vi "ReadXmlFile.vi"() -> ()   [LabVIEW 2018]
uses:
  <vilib>/xml/Load XML File.vi
  <vilib>/xml/Close Reference(Node).vi
  <vilib>/xml/NI_XML.lvlib
panel:
  out "数组":string[](array[string])
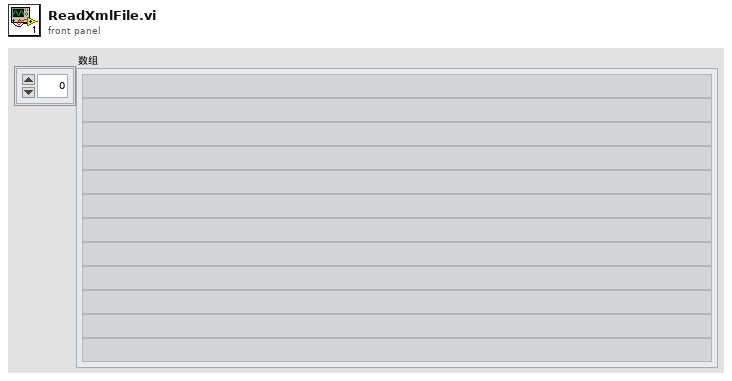
[diagram p1: front panel]
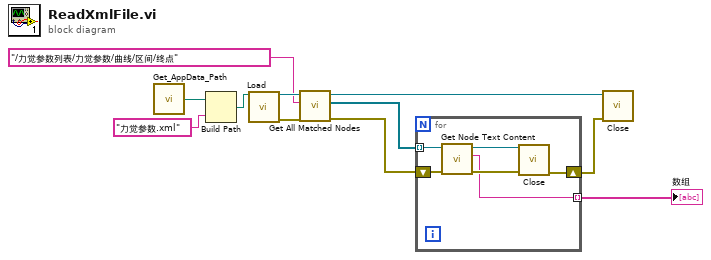
[diagram p0: block diagram]
diagram:
  n1 = call "Get_AppData_Path.vi"() -> ("path"=w7:path)  [unwired: 1 in]
  n2 = Build Path(base path=w7, name or relative path="力觉参数.xml") -> (appended path=w5:path)
  n3 = call-poly <vilib>:"Load.vi"("path to XML document"=w5) -> ("DOM document out"=w11:refnum<k20>, "error out"=w3:errorcluster)  [unwired: 12 in, 1 out]
  n4 = call <vilib>:"Get All Matched Nodes.vi"("error in (no error)"=w3, "XPath expression"="/力觉参数列表/力觉参数/曲线/区间/终点", "node in"=w11) -> ("error out"=w2:errorcluster, "node result array"=w9:refnum<k20>[], "node out"=w10:refnum<k20>)  [unwired: 6 in]
  n5 = for {
    tunnel: w9 -> [w17] mode=indexing
    tunnel: [w14] -> w8 mode=indexing
    shift-right: [w12] -> w1
    shift-left: w2 -> [w13]
    n6 = call <vilib>:"Get Node Text Content.vi"("error in (no error)"=w13, "node in"=w17) -> ("error out"=w15:errorcluster, "node text"=w14:string, "node out"=w16:refnum<k20>)  [unwired: 7 in]
    n7 = call-poly <vilib>:"Close.vi"("error in (no error)"=w15, "node"=w16) -> ("error out"=w12:errorcluster)  [unwired: 7 in]
  }
  "数组" <- w8
  n8 = call-poly <vilib>:"Close.vi"("error in (no error)"=w1, "node"=w10) -> ()  [unwired: 7 in, 1 out]
